vi "Stack Control.vi"(6 "Feeder Mode Enabled":bool, 7 "override flipper":bool, 8 "Disable Stack":bool, 9 "ConveyerBelt":dbl, 10 "Eject":bool, 11 "Suck":bool) -> (0 "frisbee counter":i16, 2 "Full Stack":bool, 3 "Empty Stack":bool, 5 "Is Sucking?":bool)   [LabVIEW 2012]
uses:
  BotStatus.vi
panel:
  # "Cannon"
  # "InFlipper"
  # "FlipperAtPlace"
  # "Middle"
  # "Bottom"
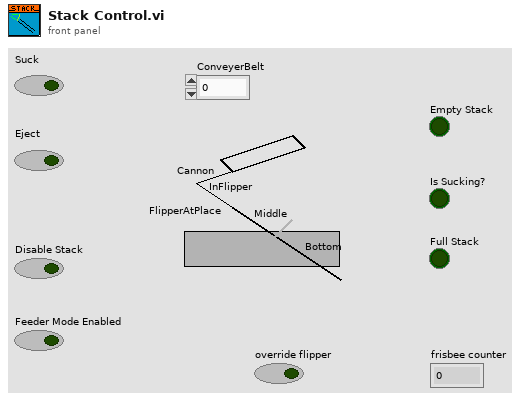
[diagram p1: front panel]
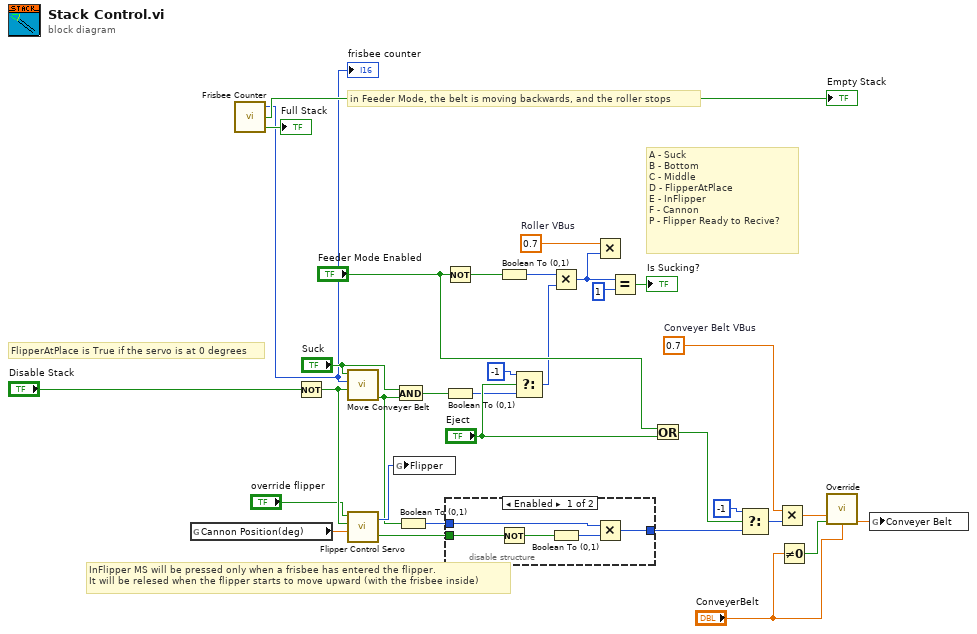
[diagram p0: block diagram]
diagram:
  w20 = 0.7  # Roller VBus
  w21 = 0.7  # Conveyer Belt VBus
  # "in Feeder Mode, the belt is moving backwards, and the roller stops"
  # "FlipperAtPlace is True if the servo is at 0 degrees"
  # "InFlipper MS will be pressed only when a frisbee has entered the flipper.\nIt will be relesed when the flipper starts to move upward (with the frisbee inside)"
  # "A - Suck\nB - Bottom\nC - Middle\nD - FlipperAtPlace\nE - InFlipper\nF - Cannon\nP - Flipper Ready to Recive?"
  n1 = global read "BotStatus.vi" "Cannon Position(deg)"() -> (w9:dbl)
  n2 = call "Frisbee Counter.vi"() -> ("frisbee counter"=w27:i16, "Stack Empty?"=→"Empty Stack":bool, "Stack Full?"=→"Full Stack":bool)  [unwired: 1 in]
  "frisbee counter" <- w27
  n3 = Not(x="Disable Stack") -> (.not. x?=w8:bool)
  n4 = call "Move Conveyer Belt.vi"("Enable Stack"=w8, "frisbee counter"=w27, "Suck"="Suck") -> ("move conveyer belt"=w5:bool)  [unwired: 6 in]
  n5 = call "Flipper Control Servo.vi"("Cannon Position(deg)"=w9, "Enable Stack"=w8, "override flipper"="override flipper") -> ("Stop Conveyer Belt"=w6:bool, "Set Flipper's Servos Angle"=w22:i32)  [unwired: 1 in]
  n6 = global write "BotStatus.vi" "Flipper"(w22) -> ()
  n7 = And(x="Suck", y=w5) -> (x .and. y?=w19:bool)
  n8 = Boolean To (0,1)(Boolean=w5) -> (0, 1=w3:i16)
  n9 = Not(x="Feeder Mode Enabled") -> (.not. x?=w11:bool)
  n10 = Boolean To (0,1)(Boolean=w19) -> (0, 1=w15:i16)
  n11 = disable-structure shown="Enabled" {
    disable-tunnel: [w34 w39] -> w2
    disable-tunnel: w3 -> [w36 w39]
    disable-tunnel: w6 -> [w38 _]
    frame Enabled {
      n12 = Not(x=w38) -> (.not. x?=w37:bool)
      n13 = Boolean To (0,1)(Boolean=w37) -> (0, 1=w35:i16)
      n14 = Multiply(x=w36, y=w35) -> (x*y=w34:i16)
    }
    frame Disabled {
    }
  }
  n15 = Boolean To (0,1)(Boolean=w11) -> (0, 1=w10:i16)
  n16 = Select(t=i16 -1, s="Eject", f=w15) -> (s? t:f=w4:i16)
  n17 = Multiply(x=w10, y=w4) -> (x*y=w7:i16)
  n18 = Multiply(x=w20, y=w7) -> ()  [unwired: 1 out]
  n19 = Equal?(x=w7, y=1) -> (x = y?=→"Is Sucking?":bool)
  n20 = Or(x="Feeder Mode Enabled", y="Eject") -> (x .or. y?=w13:bool)
  n21 = Select(t=i16 -1, s=w13, f=w2) -> (s? t:f=w17:i16)
  n22 = Multiply(x=w21, y=w17) -> (x*y=w26:dbl)
  n23 = Not Equal To 0?(x="ConveyerBelt") -> (x != 0?=w25:bool)
  n24 = call "Override.vi"("Regualer"=w26, "Override"=w25, "Overriden"="ConveyerBelt") -> ("Output"=w23:dbl)  [unwired: 12 in]
  n25 = global write "BotStatus.vi" "Conveyer Belt"(w23) -> ()
